vi "JPL Limit Control.vi"(4 "Limit Inputs":T1) -> (1 "Limit Output":cluster{"Positive Out":dbl, "Negative Out":dbl})   [LabVIEW 2014]
panel:
  out "Lower Calculation":dbl
  out "Upper Calculation":dbl
  out "Lower Limit Switch":dbl
  out "Upper Limint Switch":dbl
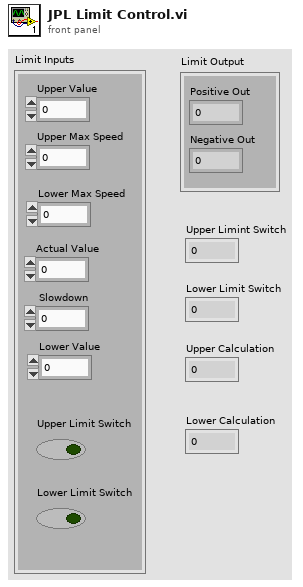
[diagram p1: front panel]
types:
  T1 = cluster{"Upper Value":dbl, "Upper Max Speed":dbl, "Actual Value":dbl, " Slowdown":dbl, "Lower Value":dbl, "Upper Limit Switch":bool, "Lower Limit Switch":bool, "Lower Max Speed":dbl}
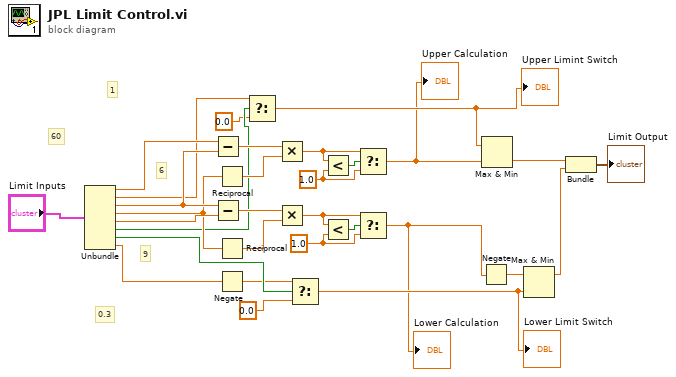
[diagram p0: block diagram]
diagram:
  w22 = 1.0
  w24 = 1.0
  # "0.3"
  # "9"
  # "6"
  # "1"
  # "60"
  n1 = Unbundle("Limit Inputs") -> ("Upper Value"=w15:dbl, "Upper Max Speed"=w5:dbl, "Actual Value"=w14:dbl, "Slowdown"=w12:dbl, "Lower Value"=w13:dbl, "Upper Limit Switch"=w6:bool, "Lower Limit Switch"=w11:bool, "Lower Max Speed"=w1:dbl)
  n2 = Subtract(x=w15, y=w14) -> (x-y=w30:dbl)
  n3 = Subtract(x=w14, y=w13) -> (x-y=w29:dbl)
  n4 = Reciprocal(x=w12) -> (1/x=w27:dbl)
  n5 = Reciprocal(x=w12) -> (1/x=w28:dbl)
  n6 = Negate(x=w1) -> (-x=w3:dbl)
  n7 = Select(t=w5, s=w6, f=0.0) -> (s? t:f=w10:dbl)
  "Upper Limint Switch" <- w10
  n8 = Multiply(x=w30, y=w27) -> (x*y=w25:dbl)
  n9 = Multiply(x=w29, y=w28) -> (x*y=w21:dbl)
  n10 = Select(t=w3, s=w11, f=0.0) -> (s? t:f=w9:dbl)
  "Lower Limit Switch" <- w9
  n11 = Less?(x=w25, y=w24) -> (x < y?=w26:bool)
  n12 = Less?(x=w21, y=w22) -> (x < y?=w23:bool)
  n13 = Select(t=w25, s=w26, f=w24) -> (s? t:f=w8:dbl)
  "Upper Calculation" <- w8
  n14 = Select(t=w21, s=w23, f=w22) -> (s? t:f=w7:dbl)
  "Lower Calculation" <- w7
  n15 = Negate(x=w7) -> (-x=w20:dbl)
  n16 = Max & Min(x=w10, y=w8) -> (min(x,y)=w18:dbl)  [unwired: 1 out]
  n17 = Max & Min(x=w20, y=w9) -> (max(x,y)=w17:dbl)  [unwired: 1 out]
  n18 = Bundle(w18, w17) -> (→"Limit Output":cluster{dbl, dbl})  [unwired: 1 in]
